vi "Trainer.vi"() -> ()   [LabVIEW 2013]
uses:
  Scanner/Database/Database.lvclass
  <instrlib>/niHWS/nihws.llb/niHWS Open File Permissions ID.ctl
  <vilib>/Analysis/5stat.llb/RMS (DBL).vi
  <vilib>/DAQmx/write.llb/DAQmx Write (Digital Bool 1Line 1Point).vi
  <vilib>/DAQmx/create/channels.llb/DAQmx Create Channel (DO-Digital Output).vi
  <instrlib>/niHWS/nihws.llb/niHWS Write Analog DBL.vi
  <vilib>/DAQmx/miscellaneous.llb/DAQmx Fill In Error Info.vi
  <vilib>/Analysis/NI_AALPro.lvlib
panel:
  in  "liquid_type":string(combo)="water"
  out "error out":errorcluster
  out "error IO":errorcluster
  in  "Rec":bool
  out "Licks":bool
  out "Last timestamp (ms)":dbl format="%#_14g"
  in  "mouse_id":dbl
  out "Delivered microL":dbl
  in  "microL/pulse":dbl=8.8
  in  "ITI":u32=500
  out "# of rewards":dbl
  in  "Calibrate":bool
  in  "Reward!":bool
  out "Water":bool
  in  "Pulse time":u32=500
  out "Correct lick":bool
  in  "% decrease Thr":dbl=10.0
  out "rms value":dbl format="%0.2f"
  out "Waveform Chart":dynamicdata(graph)
  in  "stop (F)":bool
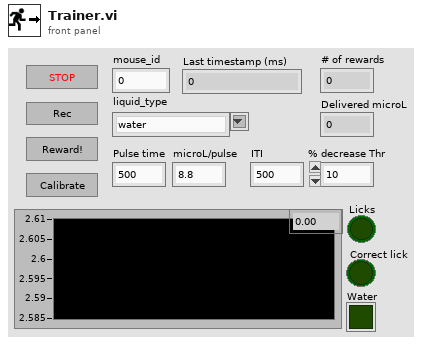
[diagram p1: front panel]
types:
  T1 = typedef "niHWS Open File Permissions ID.ctl" = enum32{"Read Only", "Read/Write Existing", "Read/Write/Create New", "Read/Write/Create New Always"}
  T2 = cluster{"mouse_id":dbl, "exp_date":string, "timestamp":dbl, "pulse_time":dbl, "microl_per_pulse":dbl, "liquid_type":string}
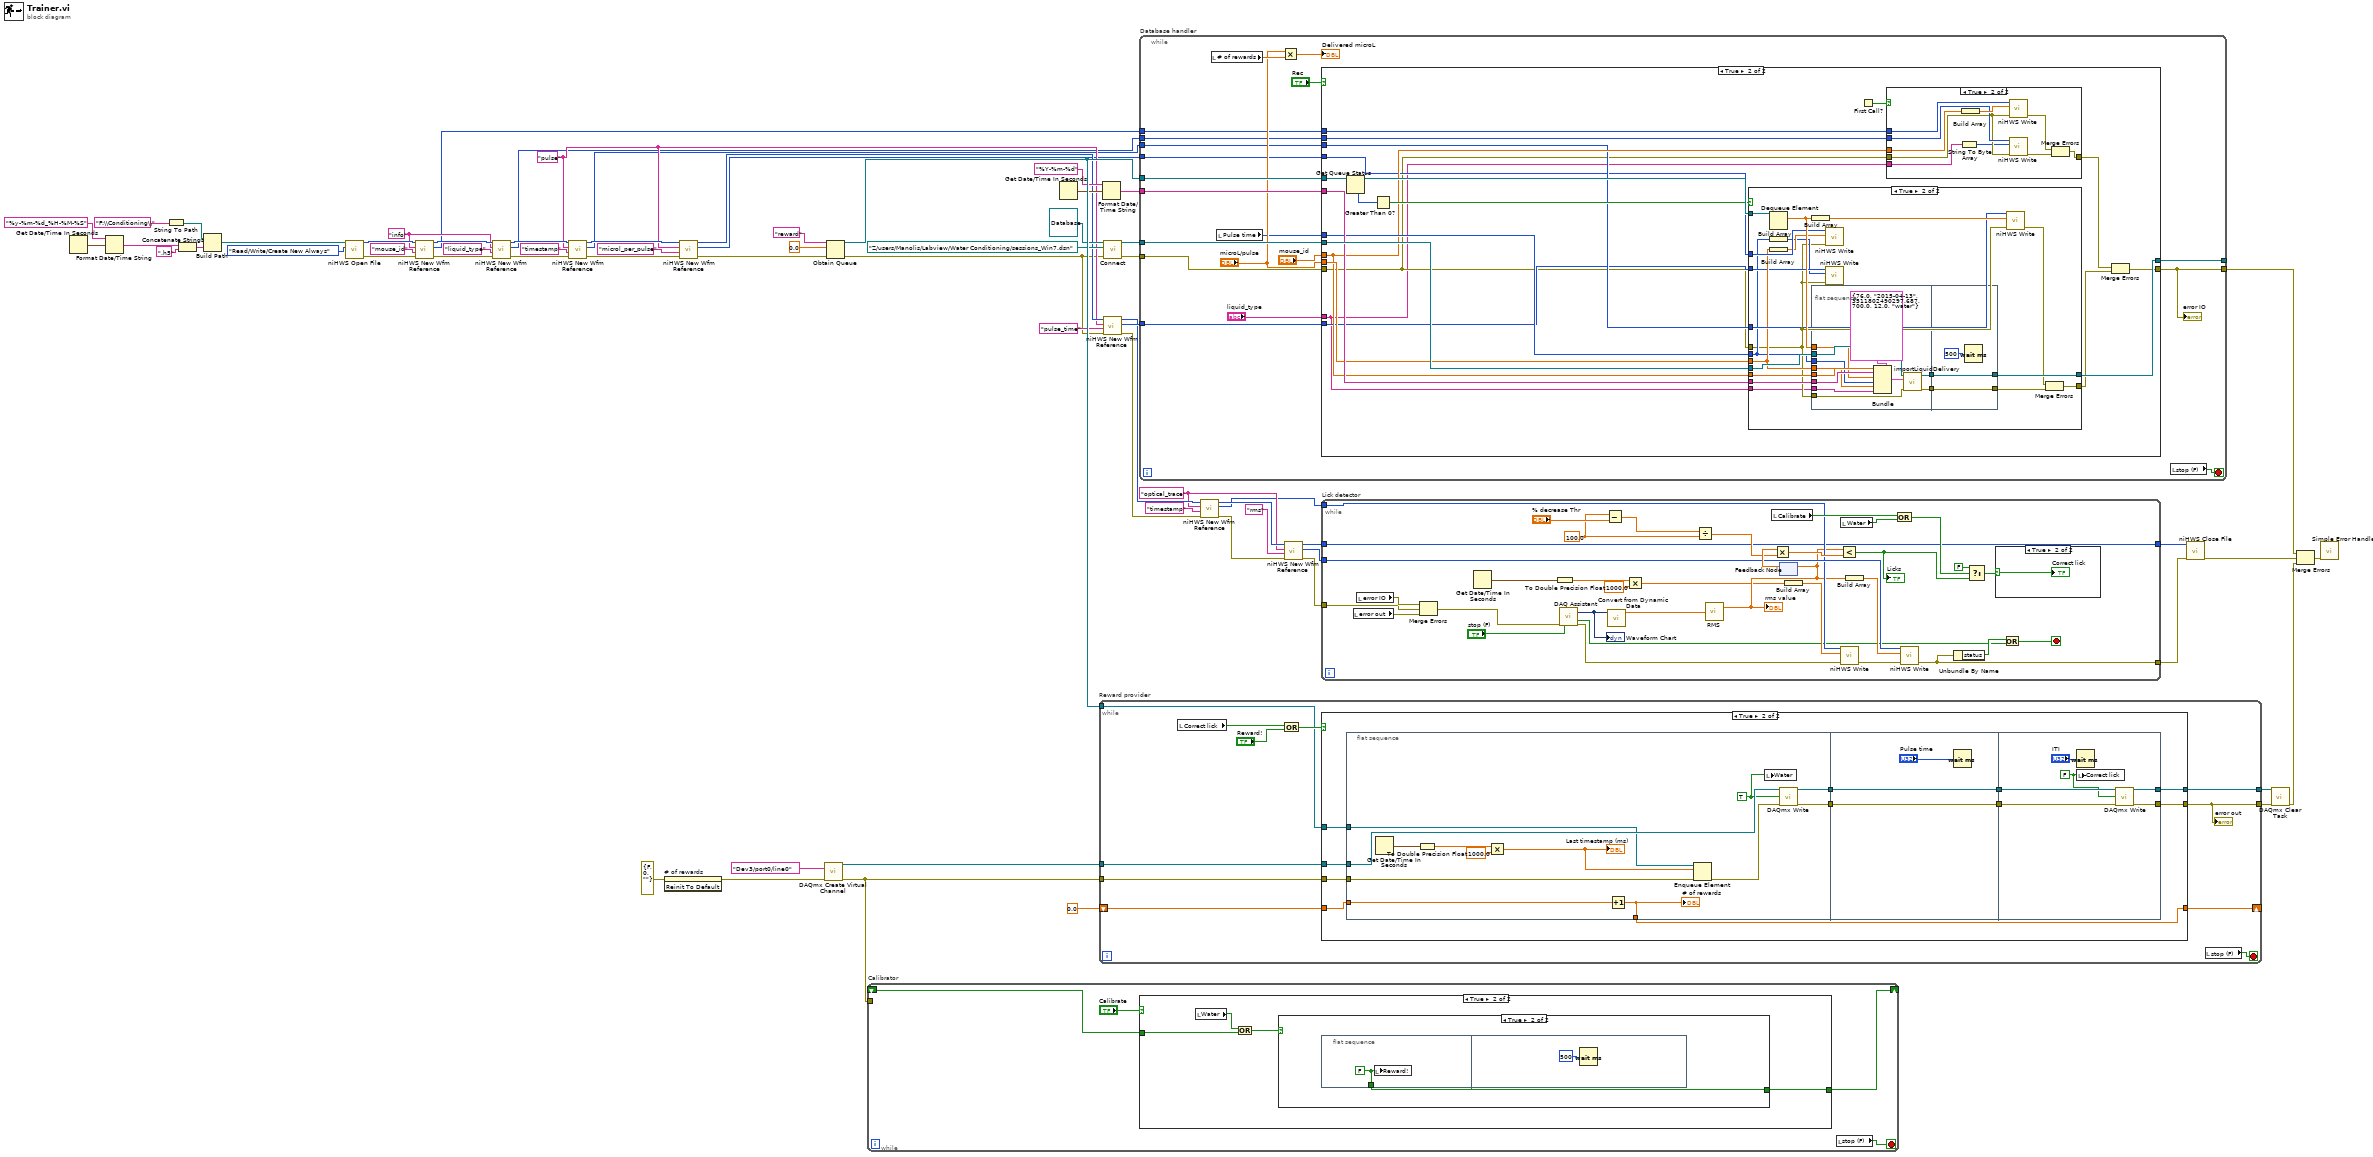
[diagram p0: block diagram]
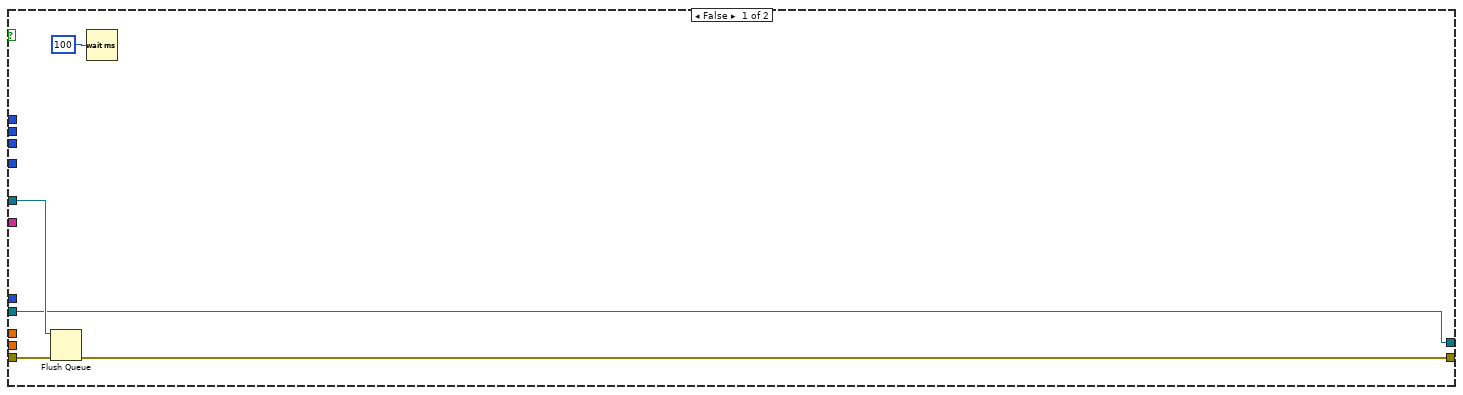
[diagram p2: hidden frame]
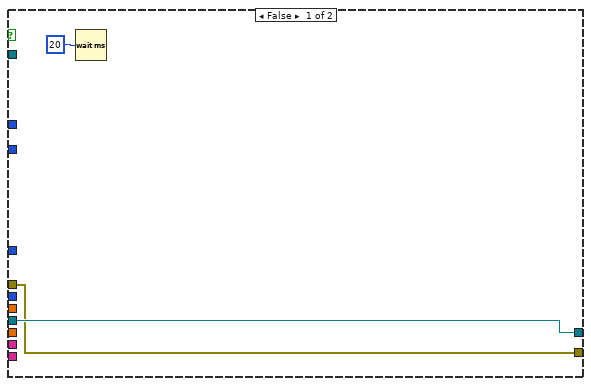
[diagram p4: hidden frame]
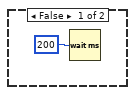
[diagram p5: hidden frame]
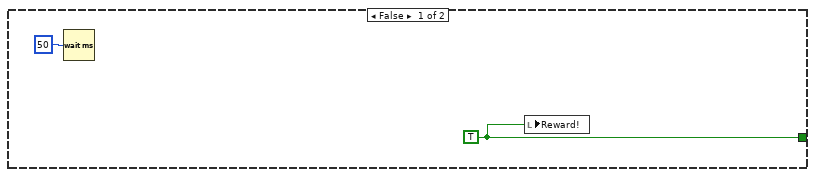
[diagram p6: hidden frame]
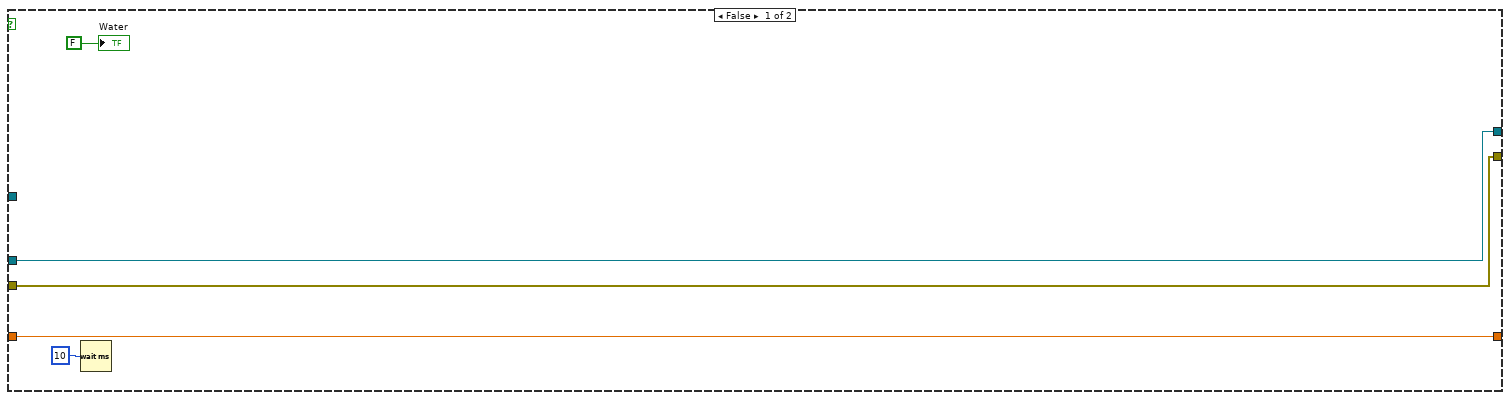
[diagram p7: hidden frame]
diagram:
  w16 = "optical_trace" ("group name (empty)")
  w27 = "pulse" ("group name (empty)")
  w36 = "info" ("group name (empty)")
  n1 = Get Date/Time In Seconds() -> (seconds since 1Jan1904=w46:timestamp)
  n2 = Format Date/Time String(time format string (%c)="%y-%m-%d_%H-%M-%S", seconds (now)=w46) -> (date/time string=w44:string)  [unwired: 1 in]
  n3 = String To Path(string="F:\\Conditioning\\" ("Default path")) -> (path=w42:path)
  n4 = Concatenate Strings(w44, ".h5" ("search string")) -> (w40:string)
  n5 = Build Path(base path=w42, name or relative path=w40) -> (appended path=w49:path)
  n6 = call <instrlib>:"niHWS Open File.vi"("permissions (0:read only)"=niHWS_Open_File_Permissions_ID."Read/Write/Create New Always", "file path"=w49) -> ("error out"=w47:errorcluster, "file handle"=w48:u32)  [unwired: 8 in]
  n7 = call <instrlib>:"niHWS New Wfm Reference.vi"("error in (no error)"=w47, "waveform name (empty)"="mouse_id", "group name (empty)"=w36, "file handle in"=w48) -> ("error out"=w38:errorcluster, "waveform reference"=w25:u32, "file handle out"=w37:u32)  [unwired: 5 in]
  n8 = call <instrlib>:"niHWS New Wfm Reference.vi"("error in (no error)"=w38, "waveform name (empty)"="liquid_type", "group name (empty)"=w36, "file handle in"=w37) -> ("error out"=w34:errorcluster, "waveform reference"=w24:u32, "file handle out"=w33:u32)  [unwired: 5 in]
  n9 = call <instrlib>:"niHWS New Wfm Reference.vi"("error in (no error)"=w34, "waveform name (empty)"="timestamp", "group name (empty)"=w27, "file handle in"=w33) -> ("error out"=w30:errorcluster, "waveform reference"=w23:u32, "file handle out"=w31:u32)  [unwired: 5 in]
  n10 = invoke on="# of rewards" class="DigNum (strict)" method="Reinit To Default"(error in=errorcluster {"status"=FALSE, "code"=0, "source"=""} ("error in (no error)")) -> (error out=w52:errorcluster)  [unwired: 2 in, 2 out]
  n11 = call <instrlib>:"niHWS New Wfm Reference.vi"("error in (no error)"=w30, "waveform name (empty)"="microl_per_pulse", "group name (empty)"=w27, "file handle in"=w31) -> ("error out"=w2:errorcluster, "waveform reference"=w22:u32, "file handle out"=w28:u32)  [unwired: 5 in]
  n12 = call-poly <vilib>:"DAQmx Create Virtual Channel.vi"("lines"=tag "Dev3/port0/line0", "error in"=w52) -> ("task out"=w66:refnum<k21>, "error out"=w9:errorcluster)  [unwired: 12 in]
  n13 = Obtain Queue(name (unnamed)="reward", element data type=0.0, error in (no error)=w2) -> (queue out=w63:refnum<queue>, error out=w1:errorcluster)  [unwired: 2 in, 1 out]
  n14 = while "Calibrator" {
    shift-right: [w70] -> _
    shift-left: _ -> [w69]
    tunnel: w9 -> [_]
    stop <- w71 stop-if-true
    n15 = case shown="True" "Calibrate" {
      tunnel: [_ w76] -> w70
      tunnel: w69 -> [_ w75]
      frame False {
        n16 = Wait (ms)(milliseconds to wait=u32 200) -> ()  [unwired: 1 out]
      }
      frame True {
        n17 = local read "Water"() -> (w73:bool)
        n18 = Or(x=w73, y=w75) -> (x .or. y?=w74:bool)
        n19 = case shown="True" w74 {
          tunnel: [w78 w79] -> w76
          frame False {
            w78 = TRUE ("Juice!")
            n20 = Wait (ms)(milliseconds to wait=u32 50) -> ()  [unwired: 1 out]
            n21 = local write "Reward!"(w78) -> ()
          }
          frame True {
            n22 = flat-sequence {
              tunnel: [w80] -> w79
              frame #0 {
                w80 = FALSE
                n23 = local write "Reward!"(w80) -> ()
              }
              frame #1 {
                n24 = Wait (ms)(milliseconds to wait=u32 500 ("value")) -> ()  [unwired: 1 out]
              }
            }
          }
        }
      }
    }
    n25 = local read "stop (F)"() -> (w71:bool)
  }
  n26 = Get Date/Time In Seconds() -> (seconds since 1Jan1904=w59:timestamp)
  n27 = while "Reward provider" {
    tunnel: w66 -> [w91]
    tunnel: [w90] -> w65
    tunnel: w9 -> [w86]
    tunnel: [w82] -> w64
    tunnel: w63 -> [w85]
    shift-right: [w84] -> _
    shift-left: 0.0 -> [w83]
    stop <- w92 stop-if-true
    n28 = local read "Correct lick"() -> (w89:bool)
    n29 = Compound Arithmetic op=OR(w89, "Reward!") -> (w88:bool)
    n30 = case shown="True" w88 {
      tunnel: w91 -> [w95 w108]
      tunnel: [w95 w107] -> w90
      tunnel: w86 -> [w94 w104]
      tunnel: [w94 w101] -> w82
      tunnel: w85 -> [_ w100]
      tunnel: w83 -> [w93 w99]
      tunnel: [w93 w98] -> w84
      frame False {
        n31 = Wait (ms)(milliseconds to wait=u32 10) -> ()  [unwired: 1 out]
        "Water" <- FALSE ("data")
      }
      frame True {
        n32 = flat-sequence {
          tunnel: w108 -> [w121]
          tunnel: [w120] -> w106
          tunnel: w104 -> [w110]
          tunnel: [w118] -> w102
          tunnel: w100 -> [w117]
          tunnel: w99 -> [w112]
          tunnel: [w111] -> w98
          tunnel: w106 -> [w123]
          tunnel: [w123] -> w105
          tunnel: [w122] -> w103
          tunnel: w102 -> [w122]
          tunnel: [w129] -> w107
          tunnel: w105 -> [w130]
          tunnel: w103 -> [w127]
          tunnel: [w126] -> w101
          frame #0 {
            w119 = TRUE ("data")
            n33 = Get Date/Time In Seconds() -> (seconds since 1Jan1904=w116:timestamp)
            n34 = To Double Precision Float(number=w116) -> (double precision float=w115:dbl)
            n35 = Multiply(x=w115, y=1000.0) -> (x*y=w113:dbl)
            "Last timestamp (ms)" <- w113
            n36 = Increment(x=w112) -> (x+1=w111:dbl)
            "# of rewards" <- w111
            n37 = Enqueue Element(queue=w117, element=w113, error in (no error)=w110) -> (error out=w109:errorcluster)  [unwired: 1 in, 2 out]
            n38 = local write "Water"(w119) -> ()
            n39 = call-poly <vilib>:"DAQmx Write.vi"("task/channels in"=w121, "data"=w119, "error in"=w109) -> ("task out"=w120:refnum<k21>, "error out"=w118:errorcluster)  [unwired: 10 in, 1 out]
          }
          frame #1 {
            n40 = Wait (ms)(milliseconds to wait="Pulse time") -> ()  [unwired: 1 out]
          }
          frame #2 {
            w125 = FALSE ("data")
            n41 = Wait (ms)(milliseconds to wait="ITI") -> ()  [unwired: 1 out]
            n42 = local write "Correct lick"(w125) -> ()
            n43 = call-poly <vilib>:"DAQmx Write.vi"("task/channels in"=w130, "data"=w125, "error in"=w127) -> ("task out"=w129:refnum<k21>, "error out"=w126:errorcluster)  [unwired: 10 in, 1 out]
          }
        }
      }
    }
    "error out" <- w82
    n44 = local read "stop (F)"() -> (w92:bool)
  }
  n45 = Format Date/Time String(time format string (%c)="%Y-%m-%d", seconds (now)=w59) -> (date/time string=w56:string)  [unwired: 1 in]
  n46 = call <instrlib>:"niHWS New Wfm Reference.vi"("error in (no error)"=w1, "waveform name (empty)"="pulse_time", "group name (empty)"=w27, "file handle in"=w28) -> ("error out"=w19:errorcluster, "waveform reference"=w21:u32, "file handle out"=w20:u32)  [unwired: 5 in]
  n47 = call-dynamic "Connect.vi"("error in (no error)"=w1, "Session"=path "Z:/users/Manolis/Labview/Water Conditioning/sessions_Win7.dsn", "Database in"=refnum<class "Database.lvclass"> refnum) -> ("error out"=w57:errorcluster, "Database out"=w58:refnum<class "Database.lvclass">)  [unwired: 7 in]
  n48 = while "Database handler" {
    tunnel: w58 -> [w148]
    tunnel: w57 -> [w146]
    tunnel: [w147] -> _
    tunnel: [w132] -> w6
    tunnel: w56 -> [w145]
    tunnel: w63 -> [w144]
    tunnel: w25 -> [w137]
    tunnel: w24 -> [w136]
    tunnel: w23 -> [w135]
    tunnel: w22 -> [w134]
    tunnel: w21 -> [w133]
    stop <- w149 stop-if-true
    n49 = local read "# of rewards"() -> (w142:dbl)
    n50 = local read "Pulse time"() -> (w139:u32)
    n51 = Multiply(x="microL/pulse", y=w142) -> (x*y=→"Delivered microL":dbl)
    n52 = case shown="True" "Rec" {
      tunnel: w148 -> [w152 w175]
      tunnel: [w152 w174] -> w147
      tunnel: [w150 w157] -> w132
      tunnel: w146 -> [w151 w159]
      tunnel: w145 -> [_ w173]
      tunnel: w144 -> [w154 w169]
      tunnel: "microL/pulse" -> [_ w168]
      tunnel: "mouse_id" -> [_ w164]
      tunnel: w139 -> [_ w167]
      tunnel: w137 -> [_ w165]
      tunnel: w136 -> [_ w163]
      tunnel: w135 -> [_ w162]
      tunnel: w134 -> [_ w161]
      tunnel: w133 -> [_ w160]
      tunnel: "liquid_type" -> [_ w155]
      frame False {
        n53 = Flush Queue(queue=w154, error in (no error)=w151) -> (error out=w150:errorcluster)  [unwired: 2 out]
        n54 = Wait (ms)(milliseconds to wait=u32 100) -> ()  [unwired: 1 out]
      }
      frame True {
        n55 = Get Queue Status(queue=w169) -> (queue out=w172:refnum<queue>, # elements in queue=w171:i32)  [unwired: 2 in, 6 out]
        n56 = Greater Than 0?(x=w171) -> (x > 0?=w170:bool)
        n57 = case shown="True" w170 {
          tunnel: w175 -> [w189 w210]
          tunnel: [w189 w209] -> w174
          tunnel: [w187 w192] -> w156
          tunnel: w159 -> [w187 w191]
          tunnel: w173 -> [_ w208]
          tunnel: w168 -> [_ w198]
          tunnel: w172 -> [_ w204]
          tunnel: w164 -> [_ w205]
          tunnel: w167 -> [_ w195]
          tunnel: w162 -> [_ w201]
          tunnel: w161 -> [_ w200]
          tunnel: w160 -> [_ w197]
          tunnel: w155 -> [_ w190]
          frame False {
            n58 = Wait (ms)(milliseconds to wait=u32 20) -> ()  [unwired: 1 out]
          }
          frame True {
            n59 = Dequeue Element(queue=w204) -> (element=w203:dbl)  [unwired: 2 in, 3 out]
            n60 = Build Array(w195) -> (w196:u32[])
            n61 = Build Array(w198) -> (w199:dbl[])
            n62 = Build Array(w203) -> (w202:dbl[])
            n63 = flat-sequence {
              tunnel: w210 -> [w222]
              tunnel: w191 -> [w219]
              tunnel: w208 -> [w216]
              tunnel: w198 -> [w213]
              tunnel: [w221] -> w207
              tunnel: [w220] -> w206
              tunnel: w205 -> [w217]
              tunnel: w195 -> [w214]
              tunnel: w203 -> [w215]
              tunnel: w190 -> [w212]
              tunnel: [w224] -> w193
              tunnel: [w225] -> w209
              tunnel: w207 -> [w225]
              tunnel: w206 -> [w224]
              frame #0 {
                n64 = Bundle(cluster=T2 {"mouse_id"=76.0, "exp_date"="2015-04-13", "timestamp"=3511802490297.687, "pulse_time"=700.0, "microl_per_pulse"=12.0, "liquid_type"="water"} ("Tuple"), "mouse_id"=w217, "exp_date"=w216, "timestamp"=w215, "pulse_time"=w214, "microl_per_pulse"=w213, "liquid_type"=w212) -> (w211:T2)
                n65 = call-dynamic "importLiquidDelivery.vi"("error in (no error)"=w219, "Tuple"=w211, "Database in"=w222) -> ("error out"=w220:errorcluster, "Database out"=w221:refnum<class "Database.lvclass">)  [unwired: 7 in]
              }
              frame #1 {
                n66 = Wait (ms)(milliseconds to wait=u32 500) -> ()  [unwired: 1 out]
              }
            }
            n67 = call-poly <instrlib>:"niHWS Write.vi"("error in (no error)"=w191, "data"=w199, "waveform reference in"=w200) -> ()  [unwired: 7 in, 2 out]
            n68 = call-poly <instrlib>:"niHWS Write.vi"("error in (no error)"=w191, "data"=w196, "waveform reference in"=w197) -> ()  [unwired: 7 in, 2 out]
            n69 = call-poly <instrlib>:"niHWS Write.vi"("error in (no error)"=w191, "data"=w202, "waveform reference in"=w201) -> ("error out"=w194:errorcluster)  [unwired: 7 in, 1 out]
            n70 = Merge Errors(w194, w193) -> (w192:errorcluster)
          }
        }
        n71 = First Call?() -> (First Call?: T/F=w166:bool)
        n72 = case shown="True" w166 {
          tunnel: w165 -> [_ w186]
          tunnel: w164 -> [_ w184]
          tunnel: w163 -> [_ w183]
          tunnel: w159 -> [w176 w182]
          tunnel: [w176 w179] -> w158
          tunnel: w155 -> [_ w178]
          frame False {
          }
          frame True {
            n73 = String To Byte Array(string=w178) -> (unsigned byte array=w177:u8[])
            n74 = Build Array(w184) -> (w185:dbl[])
            n75 = call-poly <instrlib>:"niHWS Write.vi"("error in (no error)"=w182, "data"=w185, "waveform reference in"=w186) -> ("error out"=w181:errorcluster)  [unwired: 7 in, 1 out]
            n76 = call-poly <instrlib>:"niHWS Write.vi"("error in (no error)"=w182, "data"=w177, "waveform reference in"=w183) -> ("error out"=w180:errorcluster)  [unwired: 7 in, 1 out]
            n77 = Merge Errors(w181, w180) -> (w179:errorcluster)
          }
        }
        n78 = Merge Errors(w158, w156) -> (w157:errorcluster)
      }
    }
    "error IO" <- w132
    n79 = local read "stop (F)"() -> (w149:bool)
  }
  n80 = call <instrlib>:"niHWS New Wfm Reference.vi"("error in (no error)"=w19, "waveform name (empty)"="timestamp", "group name (empty)"=w16, "file handle in"=w20) -> ("error out"=w17:errorcluster, "waveform reference"=w12:u32, "file handle out"=w18:u32)  [unwired: 5 in]
  n81 = call <instrlib>:"niHWS New Wfm Reference.vi"("error in (no error)"=w17, "waveform name (empty)"="rms", "group name (empty)"=w16, "file handle in"=w18) -> ("error out"=w8:errorcluster, "waveform reference"=w13:u32, "file handle out"=w11:u32)  [unwired: 5 in]
  n82 = while "Lick detector" {
    tunnel: w13 -> [w244]
    tunnel: w12 -> [w243]
    tunnel: w11 -> [w237]
    tunnel: [w237] -> w10
    tunnel: w8 -> [w229]
    tunnel: [w234] -> w7
    stop <- w231 stop-if-true
    w253 = 100.0 ("y")
    n83 = local read "error out"() -> (w227:errorcluster)
    n84 = local read "error IO"() -> (w230:errorcluster)
    n85 = Merge Errors(w230, w229, w227) -> (w228:errorcluster)
    n86 = Get Date/Time In Seconds() -> (seconds since 1Jan1904=w239:timestamp)
    n87 = To Double Precision Float(number=w239) -> (double precision float=w240:dbl)
    n88 = call "DAQ Assistant"("error in"=w228, "stop (F)"="stop (F)") -> ("data"=w259:dynamicdata, "stopped"=w232:bool, "error out"=w236:errorcluster)  [unwired: 14 in, 1 out]
    "Waveform Chart" <- w259
    n89 = Subtract(x=w253, y="% decrease Thr") -> (x-y=w252:dbl)
    n90 = call "Convert from Dynamic Data"("Dynamic Data Type"=w259) -> ("Array"=w258:dbl[])  [unwired: 3 in]
    n91 = Multiply(x=w240, y=1000.0) -> (x*y=w238:dbl)
    n92 = Divide(x=w252, y=w253) -> (x/y=w255:dbl)
    n93 = call-poly <vilib>:"RMS.vi"("X"=w258) -> ("rms value"=w242:dbl)  [unwired: 1 out]
    "rms value" <- w242
    n94 = local read "Calibrate"() -> (w251:bool)
    n95 = feedback #1() -> (w257:dbl)  [unwired: 1 in]
    n96 = Multiply(x=w257, y=w255) -> (x*y=w256:dbl)
    n97 = feedback-in #1(w242) -> ()
    n98 = Build Array(w238) -> (w246:dbl[])
    n99 = Less?(x=w242, y=w256) -> (x < y?=w226:bool)
    "Licks" <- w226
    n100 = local read "Water"() -> (w250:bool)
    n101 = call-poly <instrlib>:"niHWS Write.vi"("error in (no error)"=w236, "data"=w246, "waveform reference in"=w243) -> ("error out"=w235:errorcluster)  [unwired: 7 in, 1 out]
    n102 = Build Array(w242) -> (w245:dbl[])
    n103 = Compound Arithmetic op=OR(w251, w250) -> (w249:bool)
    n104 = call-poly <instrlib>:"niHWS Write.vi"("error in (no error)"=w235, "data"=w245, "waveform reference in"=w244) -> ("error out"=w234:errorcluster)  [unwired: 7 in, 1 out]
    n105 = Unbundle By Name(w234) -> ("status"=w233:bool)
    n106 = Select(t=FALSE, s=w249, f=w226) -> (s? t:f=w247:bool)
    n107 = case shown="True" w247 {
      selector: w247 -> [_ w261]
      frame False {
      }
      frame True {
        "Correct lick" <- w261
      }
    }
    n108 = Or(x=w233, y=w232) -> (x .or. y?=w231:bool)
  }
  n109 = call <instrlib>:"niHWS Close File.vi"("error in (no error)"=w7, "file handle"=w10) -> ("error out"=w5:errorcluster)  [unwired: 9 in]
  n110 = call <vilib>:"DAQmx Clear Task.vi"("task in"=w65, "error in"=w64) -> ("error out"=w4:errorcluster)  [unwired: 13 in]
  n111 = Merge Errors(w6, w5, w4) -> (w3:errorcluster)
  n112 = call <vilib>:"Simple Error Handler.vi"("error in (no error)"=w3) -> ()  [unwired: 4 in, 5 out]
